vi "GT 2D Compare Mode.vi"(8 "error in (no error)":errorcluster caption="错误输入（无错误）", 9 "mode":i16, 10 "chn":i16, 11 "cardNum":i16) -> (0 "error out":errorcluster caption="错误输出", 3 "function return":i16)   [LabVIEW 2020, in "gts.lvlib"]
doc: "GT_API GT_2DCompareMode(short cardNum,short chn,short mode);"
uses:
  gts.lvlib
  dll/32bit/multi_card/gts.dll
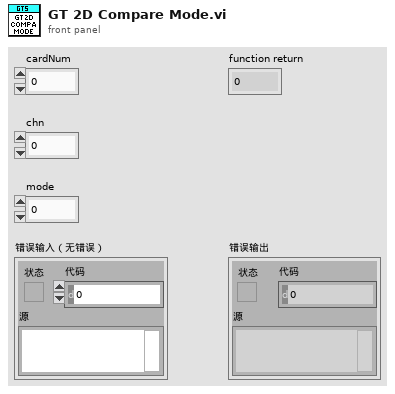
[diagram p1: front panel]
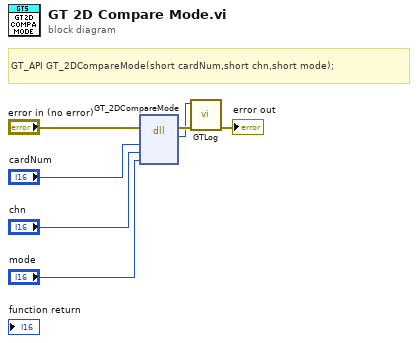
[diagram p0: block diagram]
diagram:
  # "GT_API GT_2DCompareMode(short cardNum,short chn,short mode);"
  n1 = dll-call lib="C:/1228/dll/32bit/multi_card/gts.dll" fn="GT_2DCompareMode"(error in="error in (no error)", "cardNum"="cardNum", "chn"="chn", "mode"="mode") -> (error out=w3:errorcluster, "返回类型"=w1:i16)  [unwired: 5 in, 1 out]
  n2 = call "GTLog.vi"("error in (no error)"=w3, "Numeric"=w1) -> ("error out"=→"error out":errorcluster)  [unwired: 9 in]
